vi "Get Object.vi"(8 "error in (no error)":errorcluster, 11 "Singleton in":refnum<class "Provider.lvclass">) -> (0 "error out":errorcluster, 2 "Object":refnum<class>, 3 "Singleton out":refnum<class "Provider.lvclass">)   [LabVIEW 2020, in "Provider.lvlib" / "Provider.lvclass"]
uses:
  Provider.lvclass
  Provider.lvclass/Provider.ctl
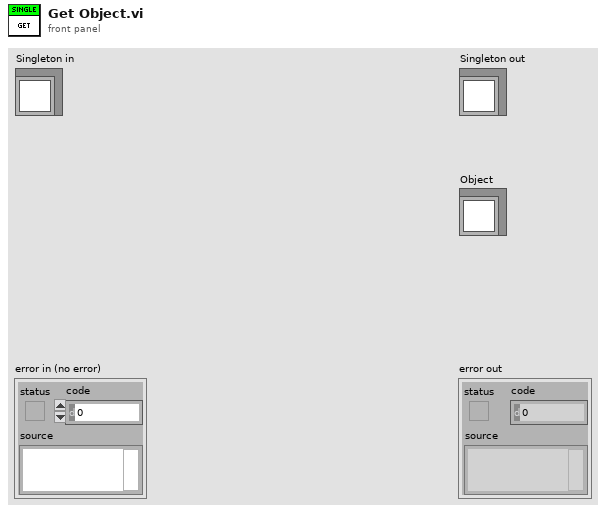
[diagram p1: front panel]
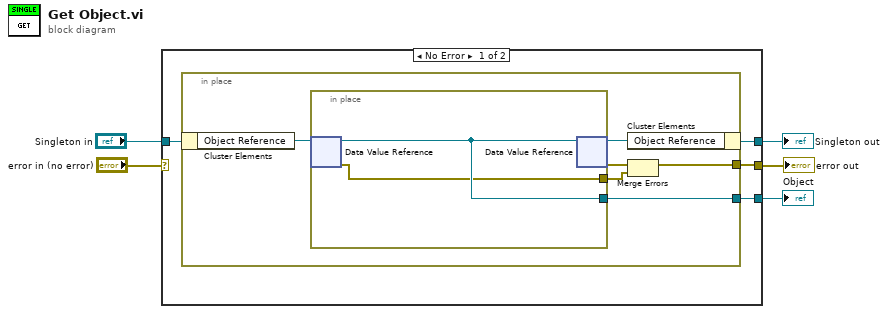
[diagram p0: block diagram]
diagram:
  n1 = case shown="No Error" "error in (no error)" {
    selector: "error in (no error)" -> [_ w19]
    tunnel: [w7 w19] -> w4
    tunnel: [w8 w18] -> w2
    tunnel: "Singleton in" -> [w9 w18]
    tunnel: [w6 _] -> w1
    frame No Error {
      n2 = in-place {
        in-place-border: [w11] -> w7
        in-place-border: [w12] -> w6
        n3 = in-place-cluster #1(w9) -> ("Object Reference"=w15:refnum<data-value>)
        n4 = in-place {
          in-place-border: [w17] -> w12
          in-place-border: [w16] -> w10
          n5 = in-place-dvr #2(w15) -> (w17:refnum<class>, w16:errorcluster)
          n6 = in-place-dvr #2(w17) -> (w14:refnum<data-value>, w13:errorcluster)
        }
        n7 = in-place-cluster #1("Object Reference"=w14) -> (w8:refnum<class "Provider.lvclass">)
        n8 = Merge Errors(w13, w10) -> (w11:errorcluster)
      }
    }
    frame Error {
    }
  }
  "error out" <- w4
  "Singleton out" <- w2
  "Object" <- w1
